vi "DDPlotter.vi"() -> ()   [LabVIEW 2021]
panel:
  in  "Relay Supply Voltage":dbl
  in  "LabJack Supply Voltage":dbl
  in  "Solenoid Supply Voltage":dbl
  in  "LS2 Flowrate":dbl
  in  "LS1 Flowrate":dbl
  in  "LP1 Engine Thrust":dbl
  in  "PT3 Pressure":dbl
  in  "PT2 Pressure":dbl
  in  "TC2 Temp":dbl
  in  "PT1 Pressure":dbl
  in  "TC1 Temp":dbl
  out "Waveform Graph":dbl[](graph)
  in  "Signals":i32(listbox)
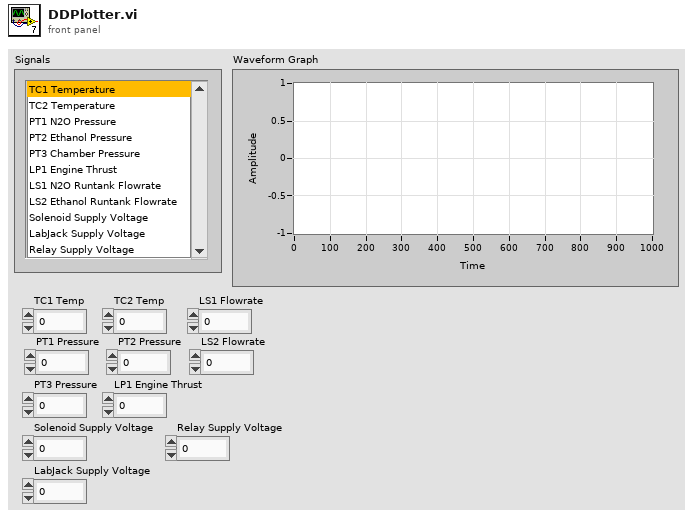
[diagram p1: front panel]
types:
  T1 = cluster{"data name":string, "drag data":variant}[]
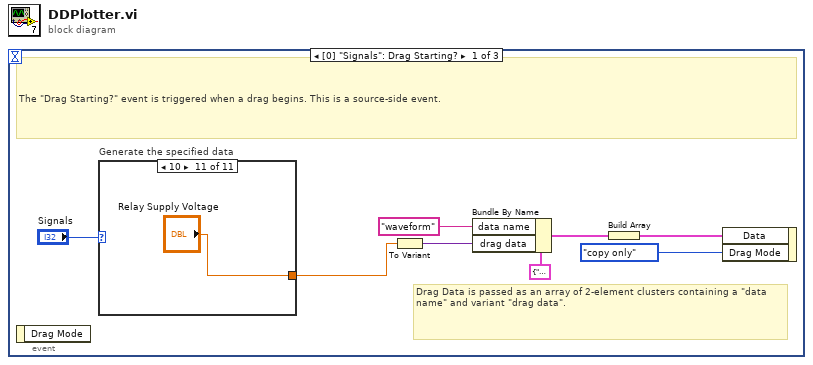
[diagram p0: block diagram]
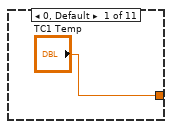
[diagram p2: hidden frame]
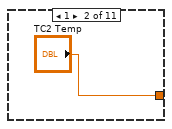
[diagram p3: hidden frame]
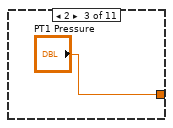
[diagram p4: hidden frame]
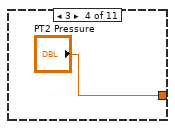
[diagram p5: hidden frame]
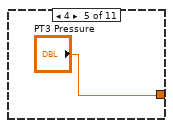
[diagram p6: hidden frame]
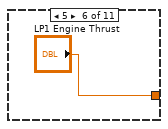
[diagram p7: hidden frame]
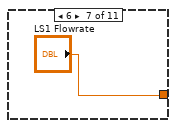
[diagram p8: hidden frame]
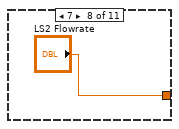
[diagram p9: hidden frame]
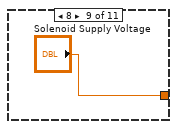
[diagram p10: hidden frame]
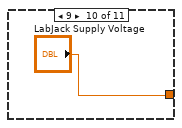
[diagram p11: hidden frame]
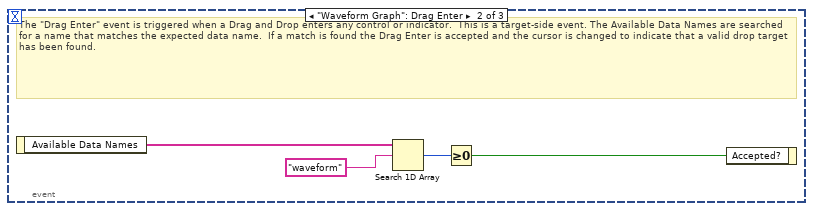
[diagram p12: hidden frame]
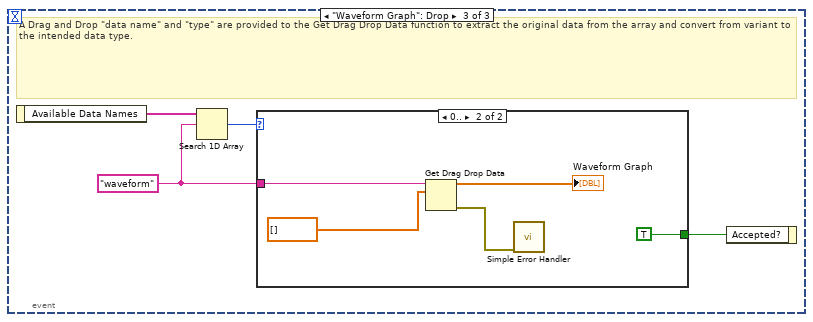
[diagram p13: hidden frame]
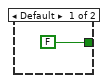
[diagram p14: hidden frame]
diagram:
  n1 = event shown="[0] \"Signals\": Drag Starting?" {
    selector: _ -> [_ _ _]
    dyn-events: _ -> [_ _ _]
    timeout: _ -> [_ _ _]
    event "Signals": Drag Starting? {
      # "Drag Data is passed as an array of 2-element clusters containing a \"data name\" and variant \"drag data\"."
      # "The \"Drag Starting?\" event is triggered when a drag begins. This is a source-side event."
      n2 = event-data() -> ()  [unwired: 1 in, 1 out]
      n3 = case "Generate the specified data" shown="10" "Signals" {
        tunnel: ["TC1 Temp" "TC2 Temp" "PT1 Pressure" "PT2 Pressure" "PT3 Pressure" "LP1 Engine Thrust" "LS1 Flowrate" "LS2 Flowrate" "Solenoid Supply Voltage" "LabJack Supply Voltage" "Relay Supply Voltage"] -> w1
        frame 0, Default {
        }
        frame 1 {
        }
        frame 2 {
        }
        frame 3 {
        }
        frame 4 {
        }
        frame 5 {
        }
        frame 6 {
        }
        frame 7 {
        }
        frame 8 {
        }
        frame 9 {
        }
        frame 10 {
        }
      }
      n4 = To Variant(anything=w1) -> (Variant=w7:variant)
      n5 = Bundle By Name(cluster=cluster{"data name":string, "drag data":variant} {"data name"="", "drag data"=variant}, "data name"="waveform", "drag data"=w7) -> (w5:cluster{"data name":string, "drag data":variant})
      n6 = Build Array(w5) -> (w4:T1)
      n7 = event-data("Data"=w4, "Drag Mode"=enum32{"copy or move", "copy only", "move only"}."copy only") -> ()  [unwired: 1 in, 1 out]
    }
    event "Waveform Graph": Drag Enter {
      # "The \"Drag Enter\" event is triggered when a Drag and Drop enters any control or indicator.  This is a target-side event. The Available Data Names are searched for a name that matches the expected data name.  If a match is found the Drag Enter is accepted and the cursor is changed to indicate that a valid drop target has been found."
      n8 = event-data() -> ("Available Data Names"=w23:string[])  [unwired: 1 in]
      n9 = Search 1D Array(1D array=w23, element="waveform") -> (index of element=w20:i32)  [unwired: 1 in]
      n10 = Greater Or Equal To 0?(x=w20) -> (x >= 0?=w21:bool)
      n11 = event-data("Accepted?"=w21) -> ()  [unwired: 1 in, 1 out]
    }
    event "Waveform Graph": Drop {
      w24 = "waveform" ("element")
      # "A Drag and Drop \"data name\" and \"type\" are provided to the Get Drag Drop Data function to extract the original data from the array and convert from variant to the intended data type."
      n12 = event-data() -> ("Available Data Names"=w27:string[])  [unwired: 1 in]
      n13 = Search 1D Array(1D array=w27, element=w24) -> (index of element=w25:i32)  [unwired: 1 in]
      n14 = case shown="0.." w25 {
        tunnel: [FALSE TRUE] -> w26
        tunnel: w24 -> [_ w29]
        frame Default {
        }
        frame 0.. {
          n15 = Get Drag Drop Data(8:dbl[] [], 9:w29) -> (0:w30:errorcluster, 3:→"Waveform Graph":dbl[])  [unwired: 1 in]
          n16 = call <vilib>:"Simple Error Handler.vi"("error in (no error)"=w30) -> ()  [unwired: 4 in, 5 out]
        }
      }
      n17 = event-data("Accepted?"=w26) -> ()  [unwired: 1 in, 1 out]
    }
  }
